vi "sub_deg-gap-cal_4_pid.vi"() -> (3 "deg gap":dbl format="%.1f")   [LabVIEW 2019]
uses:
  Ctrl/pid-in-params.ctl
  Ctrl/cmd_common.ctl
panel:
  out "distance gap":dbl format="%.1f"
  out "trans agv-c":dbl format="%.1f"
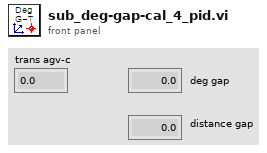
[diagram p1: front panel]
types:
  T1 = typedef "cmd_common.ctl" = enum16{"read", "write"}
  T2 = typedef "pid-in-params.ctl" = enum16{"read", "write"}
  T3 = cluster{"lookahead":cluster{"x":dbl, "y":dbl}, "looktail":cluster{"x":dbl, "y":dbl}, "lookahead circle in":cluster{"x":dbl, "y":dbl}[], "center":cluster{"x":dbl, "y":dbl}, "wpt closest":cluster{"x":dbl, "y":dbl}}
  T4 = cluster{"deg_agv-lookahead":dbl, "deg_waypoint":dbl, "deg_gap":dbl, "deg_target":dbl, "pid output":dbl, "dis-gap":dbl, "deg_agv-center":dbl}
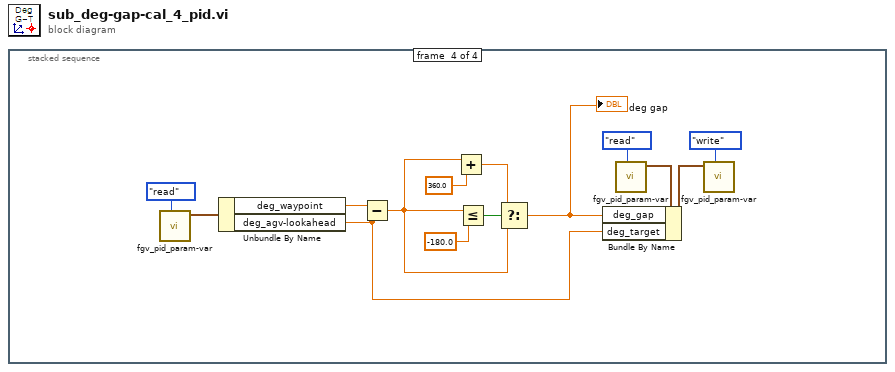
[diagram p0: block diagram]
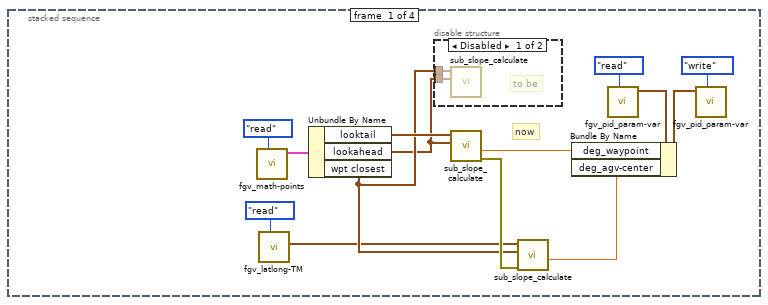
[diagram p2: hidden frame]
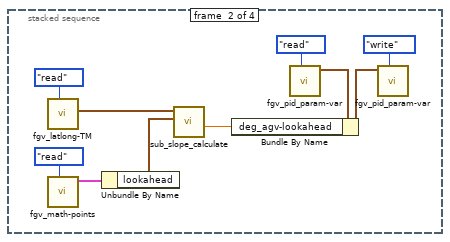
[diagram p4: hidden frame]
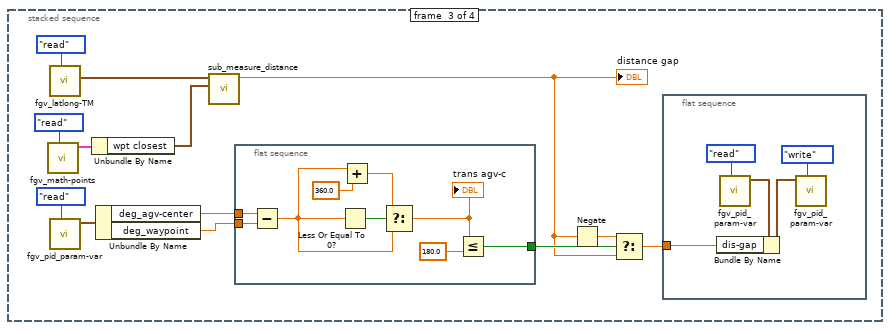
[diagram p5: hidden frame]
diagram:
  n1 = stacked-sequence {
    frame #0 {
      # "now"
      n2 = call "fgv_math-points.vi"("cmd"=cmd_common."read") -> ("point-db out"=w9:T3)  [unwired: 10 in]
      n3 = call "fgv_latlong-TM.vi"("cmd"=enum16{"write", "read"}."read") -> ("tm out"=w1:cluster{"YE":dbl, "XN":dbl})  [unwired: 9 in, 1 out]
      n4 = Unbundle By Name(w9) -> ("looktail"=w8:cluster{"x":dbl, "y":dbl}, "lookahead"=w2:cluster{"x":dbl, "y":dbl}, "wpt closest"=w3:cluster{"x":dbl, "y":dbl})
      n5 = disable-structure shown="Disabled" {
        disable-tunnel: w3 -> [w16 _]
        disable-tunnel: w2 -> [w15 _]
        frame Disabled {
          # "to be"
          n6 = call "sub_slope_calculate.vi"("point n+1"=w15, "point n"=w16) -> ()  [unwired: 7 in, 3 out]
        }
        frame Enabled {
        }
      }
      n7 = call "sub_slope_calculate.vi"("point n+1"=w2, "point n"=w8) -> ("error out"=w6:errorcluster, "deg_gps-base"=w7:dbl)  [unwired: 7 in, 1 out]
      n8 = call "sub_slope_calculate.vi"("error in"=w6, "point n+1"=w3, "point n"=w1) -> ("deg_gps-base"=w5:dbl)  [unwired: 6 in, 2 out]
      n9 = call "fgv_pid_param-var.vi"("cmd"=pid-in-params."read") -> ("pid-var_output"=w11:T4)  [unwired: 10 in]
      n10 = Bundle By Name(cluster=w11, "deg_waypoint"=w7, "deg_agv-center"=w5) -> (w12:T4)
      n11 = call "fgv_pid_param-var.vi"("cmd"=pid-in-params."write", "pid-vars_in"=w12) -> ()  [unwired: 9 in, 1 out]
    }
    frame #1 {
      n12 = call "fgv_latlong-TM.vi"("cmd"=enum16{"write", "read"}."read") -> ("tm out"=w17:cluster{"YE":dbl, "XN":dbl})  [unwired: 9 in, 1 out]
      n13 = call "fgv_math-points.vi"("cmd"=cmd_common."read") -> ("point-db out"=w21:T3)  [unwired: 10 in]
      n14 = Unbundle By Name(w21) -> ("lookahead"=w20:cluster{"x":dbl, "y":dbl})
      n15 = call "sub_slope_calculate.vi"("point n+1"=w20, "point n"=w17) -> ("deg_gps-base"=w18:dbl)  [unwired: 7 in, 2 out]
      n16 = call "fgv_pid_param-var.vi"("cmd"=pid-in-params."read") -> ("pid-var_output"=w23:T4)  [unwired: 10 in]
      n17 = Bundle By Name(cluster=w23, "deg_agv-lookahead"=w18) -> (w24:T4)
      n18 = call "fgv_pid_param-var.vi"("cmd"=pid-in-params."write", "pid-vars_in"=w24) -> ()  [unwired: 9 in, 1 out]
    }
    frame #2 {
      n19 = call "fgv_math-points.vi"("cmd"=cmd_common."read") -> ("point-db out"=w36:T3)  [unwired: 10 in]
      n20 = call "fgv_latlong-TM.vi"("cmd"=enum16{"write", "read"}."read") -> ("tm out"=w27:cluster{"YE":dbl, "XN":dbl})  [unwired: 9 in, 1 out]
      n21 = call "fgv_pid_param-var.vi"("cmd"=pid-in-params."read") -> ("pid-var_output"=w32:T4)  [unwired: 10 in]
      n22 = Unbundle By Name(w36) -> ("wpt closest"=w34:cluster{"x":dbl, "y":dbl})
      n23 = Unbundle By Name(w32) -> ("deg_agv-center"=w31:dbl, "deg_waypoint"=w30:dbl)
      n24 = call "sub_measure_distance.vi"("pt 2"=w34, "pt 1"=w27) -> ("distance"=w29:dbl)  [unwired: 9 in]
      "distance gap" <- w29
      n25 = flat-sequence {
        tunnel: [w47] -> w35
        tunnel: w31 -> [w46]
        tunnel: w30 -> [w45]
        frame #0 {
          n26 = Subtract(x=w46, y=w45) -> (x-y=w50:dbl)
          n27 = Less Or Equal To 0?(x=w50) -> (x <= 0?=w53:bool)
          n28 = Add(x=w50, y=360.0) -> (x+y=w51:dbl)
          n29 = Select(t=w51, s=w53, f=w50) -> (s? t:f=w49:dbl)
          "trans agv-c" <- w49
          n30 = Less Or Equal?(x=w49, y=180.0) -> (x <= y?=w47:bool)
        }
      }
      n31 = Negate(x=w29) -> (-x=w39:dbl)
      n32 = Select(t=w39, s=w35, f=w29) -> (s? t:f=w37:dbl)
      n33 = flat-sequence {
        tunnel: w37 -> [w40]
        frame #0 {
          n34 = call "fgv_pid_param-var.vi"("cmd"=pid-in-params."read") -> ("pid-var_output"=w42:T4)  [unwired: 10 in]
          n35 = Bundle By Name(cluster=w42, "dis-gap"=w40) -> (w41:T4)
          n36 = call "fgv_pid_param-var.vi"("cmd"=pid-in-params."write", "pid-vars_in"=w41) -> ()  [unwired: 9 in, 1 out]
        }
      }
    }
    frame #3 {
      n37 = call "fgv_pid_param-var.vi"("cmd"=pid-in-params."read") -> ("pid-var_output"=w66:T4)  [unwired: 10 in]
      n38 = Unbundle By Name(w66) -> ("deg_waypoint"=w65:dbl, "deg_agv-lookahead"=w54:dbl)
      n39 = Subtract(x=w65, y=w54) -> (x-y=w59:dbl)
      n40 = Add(x=w59, y=360.0) -> (x+y=w56:dbl)
      n41 = Less Or Equal?(x=w59, y=-180.0) -> (x <= y?=w58:bool)
      n42 = Select(t=w56, s=w58, f=w59) -> (s? t:f=w55:dbl)
      "deg gap" <- w55
      n43 = call "fgv_pid_param-var.vi"("cmd"=pid-in-params."read") -> ("pid-var_output"=w63:T4)  [unwired: 10 in]
      n44 = Bundle By Name(cluster=w63, "deg_gap"=w55, "deg_target"=w54) -> (w62:T4)
      n45 = call "fgv_pid_param-var.vi"("cmd"=pid-in-params."write", "pid-vars_in"=w62) -> ()  [unwired: 9 in, 1 out]
    }
  }
